vi "Configure Global Settings.vi"(7 "Enable Global Output (F: Disable)":bool, 8 "error in (no error)":errorcluster, 9 "Global Current (0)":dbl, 10 "Global Voltage (0)":dbl, 11 "VISA resource name":refnum<visa-resource-name>) -> (0 "error out":errorcluster, 3 "VISA resource name out":refnum<visa-resource-name>)   [LabVIEW 2023]
doc: "Configures the voltage, current and output for all channels in a multi-channel system."
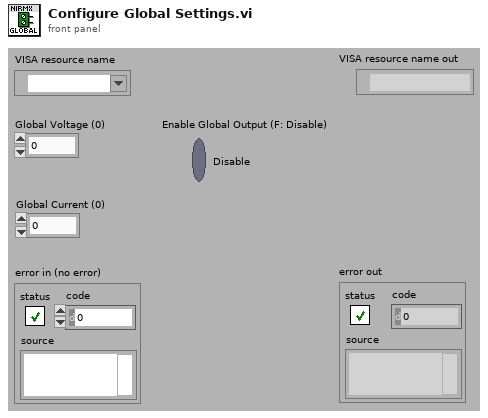
[diagram p1: front panel]
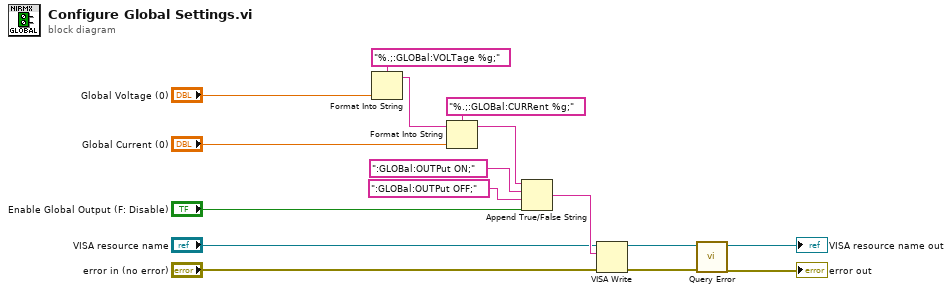
[diagram p0: block diagram]
diagram:
  n1 = Format Into String(format string="%.;:GLOBal:VOLTage %g;", "Global Voltage (0)") -> (resulting string=w14:string)  [unwired: 2 in, 1 out]
  n2 = Format Into String(format string="%.;:GLOBal:CURRent %g;", initial string=w14, "Global Current (0)") -> (resulting string=w11:string)  [unwired: 1 in, 1 out]
  n3 = Append True/False String(1:"Enable Global Output (F: Disable)", 2:":GLOBal:OUTPut OFF;", 3:":GLOBal:OUTPut ON;", 4:w11) -> (0:w7:string)
  n4 = VISA Write(VISA resource name="VISA resource name", write buffer=w7, error in (no error)="error in (no error)") -> (VISA resource name out=w4:refnum<visa-resource-name>, error out=w3:errorcluster)  [unwired: 1 out]
  n5 = call "Query Error.vi"("error in (no error)"=w3, "VISA resource name"=w4) -> ("error out"=→"error out":errorcluster, "VISA resource name out"=→"VISA resource name out":refnum<visa-resource-name>)  [unwired: 6 in, 2 out]
